vi "getCoolerIndicator.vi"(8 "error in (no error)":errorcluster, 11 "CameraTempController.lvclass in":refnum<class "CameraTempController.lvclass">) -> (0 "error out":errorcluster, 2 "Cooler":bool, 3 "CameraTempController.lvclass out":refnum<class "CameraTempController.lvclass">)   [LabVIEW 2011, in "Hardware.lvlib" / "Channels.lvlib" / "CameraTempController.lvclass"]
uses:
  CameraTempController.lvclass
  CameraTempController.lvclass/CameraTempController.ctl
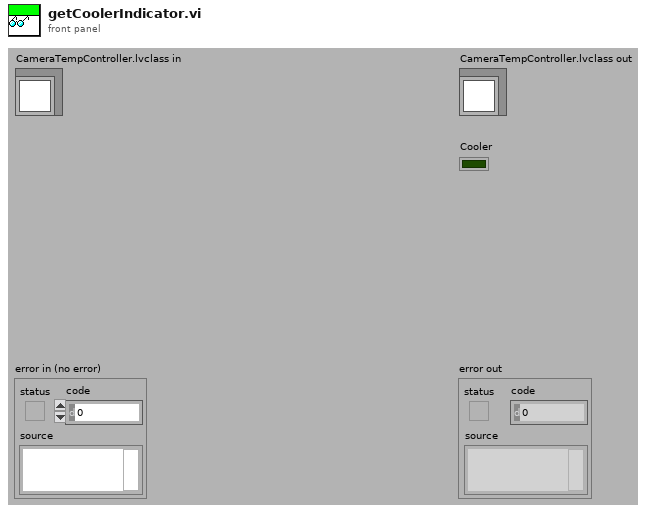
[diagram p1: front panel]
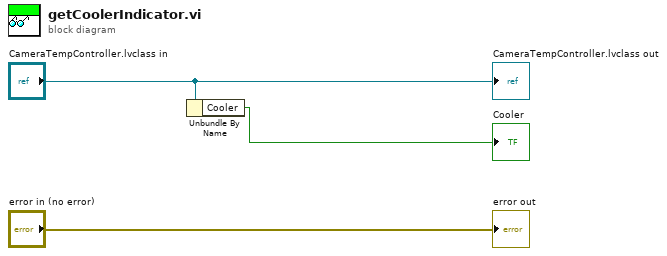
[diagram p0: block diagram]
diagram:
  n1 = Unbundle By Name("CameraTempController.lvclass in") -> ("Cooler"=→"Cooler":bool)
  "error out" <- "error in (no error)"
  "CameraTempController.lvclass out" <- "CameraTempController.lvclass in"
